vi "Actor Core.vi"(8 "error in":errorcluster, 11 "output_actor_errorneous in":refnum<class "Output Actor Hardware.lvclass">) -> (0 "error out":errorcluster, 3 "Actor out":refnum<class "Actor.lvclass">)   [LabVIEW 2015, in "Output Actor Hardware.lvclass"]
doc: "(<B>Filename</B>: Actor Framework.lvlib:Actor.lvclass:Actor Core.vi)\n\nReceives messages to the actor, reacts to them, and initiates any error handling that may shut the actor down.\n\nDescendant classes may override this VI to append parallel tasks for the actor to complete while it handles messages. Overrides use the Call Parent Method node."
uses:
  Output Actor Hardware.lvclass
  <vilib>/ActorFramework/Actor/Actor.lvclass
  state.ctl
  <vilib>/ActorFramework/Actor/Actor.lvclass/Actor.ctl
  <vilib>/ActorFramework/Message Enqueuer/Message Enqueuer.lvclass/Message Enqueuer.ctl
  Output Actor Hardware.lvclass/Output Actor Hardware.ctl
  <vilib>/ActorFramework/Message Enqueuer/Init from Existing Queue.vi
  <vilib>/ActorFramework/Message Enqueuer/Enqueue.vi
  <vilib>/ActorFramework/Message Priority Queue/Priority Enqueue.vi
  <vilib>/ActorFramework/Message Enqueuer/Message Enqueuer.lvclass
  Output Actor Hardware Messages/Do Check Available Msg/Do Check Available Msg.lvclass
  Output Actor Hardware Messages/Do Check Still Available Msg/Do Check Still Available Msg.lvclass
  output actor/Output Actor.lvclass
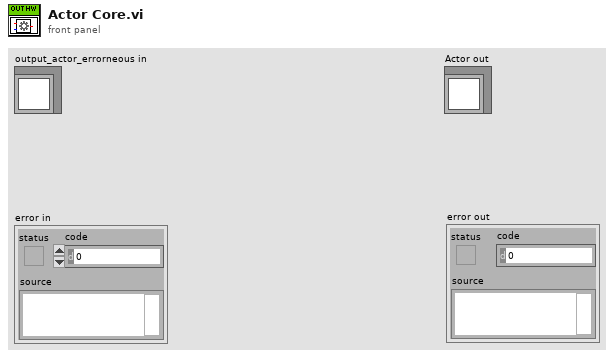
[diagram p1: front panel]
types:
  T1 = typedef "Output Actor Hardware.lvclass/state.ctl" = enum16{"not_available", "not_initialized", "ok"}
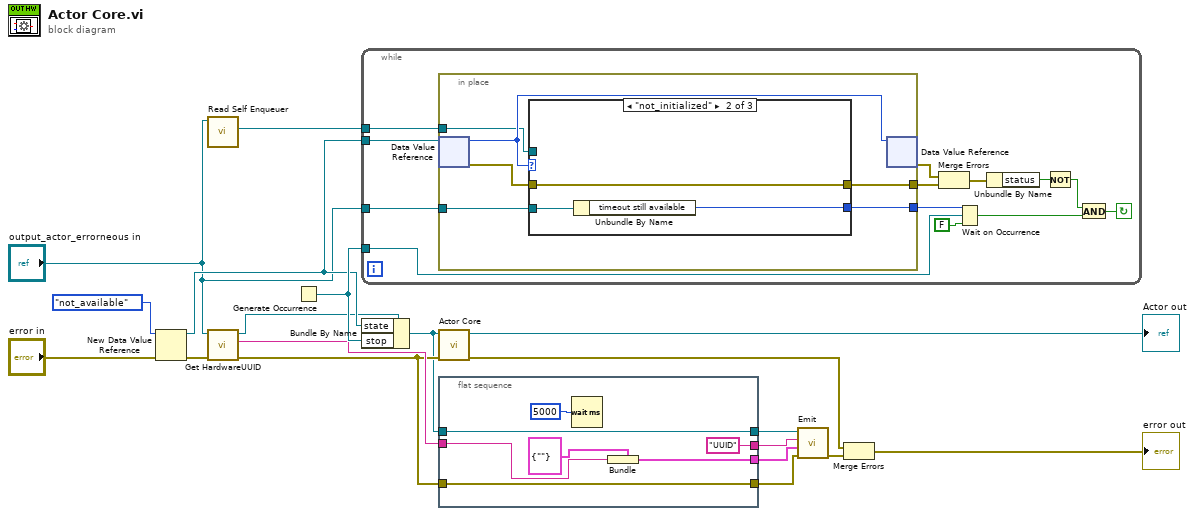
[diagram p0: block diagram]
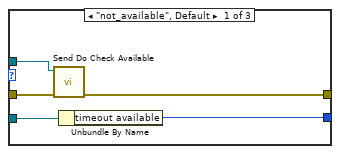
[diagram p2: hidden frame]
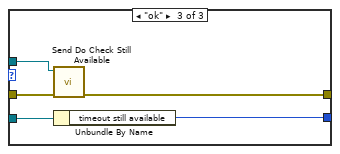
[diagram p3: hidden frame]
diagram:
  n1 = New Data Value Reference(data value=state."not_available" ("state"), error in="error in") -> (data value reference=w14:refnum<data-value>, error out=w13:errorcluster)
  n2 = call <vilib>:"Read Self Enqueuer.vi"("Actor"="output_actor_errorneous in") -> ("Self Enqueuer"=w16:refnum<class "Message Enqueuer.lvclass">)  [unwired: 10 in]
  n3 = call "Get HardwareUUID.vi"("error in (no error)"=w13, "Output Actor Hardware in"="output_actor_errorneous in") -> ("error out"=w7:errorcluster, "UUID"=w11:string, "Output Actor Hardware out"=w2:refnum<class "Output Actor Hardware.lvclass">)  [unwired: 7 in]
  n4 = Generate Occurrence() -> (w15:refnum<k4>)
  n5 = while {
    tunnel: w14 -> [w32]
    tunnel: w15 -> [w30]
    tunnel: w16 -> [w29]
    tunnel: "output_actor_errorneous in" -> [w27]
    stop <- w20 continue-if-true
    n6 = in-place {
      in-place-border: w29 -> [w37]
      in-place-border: [w35] -> w28
      in-place-border: w27 -> [w34]
      in-place-border: [w33] -> w25
      n7 = in-place-dvr #1(w32) -> (w38:T1, w36:errorcluster)
      n8 = case shown="\"not_initialized\"" w38 {
        tunnel: w37 -> [w43 _ w51]
        tunnel: w36 -> [w42 w44 w50]
        tunnel: [w40 w45 w48] -> w35
        tunnel: w34 -> [w41 w46 w49]
        tunnel: [w39 w44 w47] -> w33
        frame "not_available", Default {
          n9 = call "Send Do Check Available.vi"("error in (no error)"=w42, "Message Enqueuer"=w43) -> ("error out"=w39:errorcluster)  [unwired: 8 in, 1 out]
          n10 = Unbundle By Name(w41) -> ("timeout available"=w40:i32)
        }
        frame "not_initialized" {
          n11 = Unbundle By Name(w46) -> ("timeout still available"=w45:i32)
        }
        frame "ok" {
          n12 = call "Send Do Check Still Available.vi"("error in (no error)"=w50, "Message Enqueuer"=w51) -> ("error out"=w47:errorcluster)  [unwired: 8 in, 1 out]
          n13 = Unbundle By Name(w49) -> ("timeout still available"=w48:i32)
        }
      }
      n14 = in-place-dvr #1(w38) -> (w26:errorcluster)  [unwired: 1 out]
    }
    n15 = Merge Errors(w26, w25) -> (w24:errorcluster)
    n16 = Wait on Occurrence(1:FALSE ("ignore previous (T)"), 2:w30, 3:w28) -> (0:w21:bool)
    n17 = Unbundle By Name(w24) -> ("status"=w22:bool)
    n18 = Not(x=w22) -> (.not. x?=w23:bool)
    n19 = And(x=w23, y=w21) -> (x .and. y?=w20:bool)
  }
  n20 = Bundle By Name(cluster=w2, "state"=w14, "stop"=w15) -> (w1:refnum<class "Output Actor Hardware.lvclass">)
  n21 = call-parent "Actor Core.vi"("error in"=w7, "output_actor in"=w1) -> ("error out"=w4:errorcluster, "Actor out"=→"Actor out":refnum<class "Actor.lvclass">)  [unwired: 8 in]
  n22 = flat-sequence {
    tunnel: w11 -> [w55]
    tunnel: w1 -> [w57]
    tunnel: [w57] -> w10
    tunnel: [w54] -> w9
    tunnel: ["UUID" ("function")] -> w8
    tunnel: w7 -> [w52]
    tunnel: [w52] -> w6
    frame #0 {
      n23 = Wait (ms)(milliseconds to wait=u32 5000) -> ()  [unwired: 1 out]
      n24 = Bundle(cluster=cluster{"UUID":string} {"UUID"=""}, "UUID"=w55) -> (w54:cluster{"UUID":string})
    }
  }
  n25 = call "Emit.vi"("error in (no error)"=w6, "parameter"=w9, "function"=w8, "output_actor in"=w10) -> ("error out"=w5:errorcluster)  [unwired: 6 in, 1 out]
  n26 = Merge Errors(w4, w5) -> (→"error out":errorcluster)
